vi "Read filename.vi"(8 "error in (no error)":errorcluster, 11 "file attributes in":refnum<class "File Attributes.lvclass">) -> (0 "error out":errorcluster, 2 "filename":string, 3 "file attributes out":refnum<class "File Attributes.lvclass">)   [LabVIEW 2020, in "NI_SFTP.lvlib" / "File Attributes.lvclass"]
doc: "Reads the filename stored in this File Attributes object.\n\nThis property may not always be populated by SFTP VIs. If it does not exist, an error is returned."
uses:
  <vilib>/net/SFTP/File Attributes/File Attributes.lvclass
  <vilib>/net/SFTP/File Attributes/File Attributes.lvclass/File Attributes.ctl
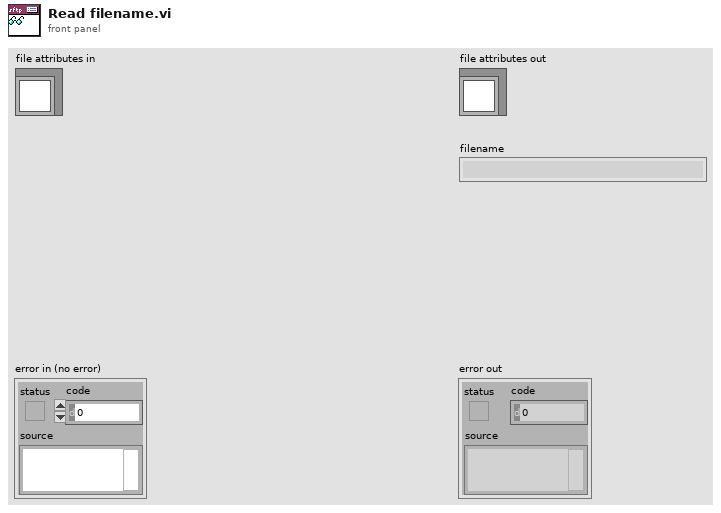
[diagram p1: front panel]
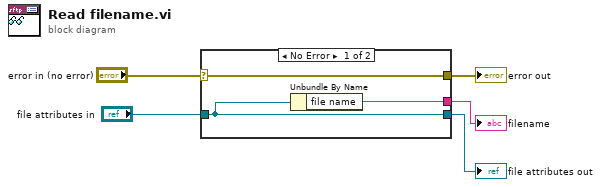
[diagram p0: block diagram]
diagram:
  n1 = case shown="No Error" "error in (no error)" {
    selector: "error in (no error)" -> [w8 w9]
    tunnel: [w8 w9] -> w4
    tunnel: [w7 w10] -> w2
    tunnel: "file attributes in" -> [w7 w10]
    tunnel: [w6 _] -> w1
    frame No Error {
      n2 = Unbundle By Name(w7) -> ("file name"=w6:string)
    }
    frame Error {
    }
  }
  "error out" <- w4
  "file attributes out" <- w2
  "filename" <- w1
